vi "findNewLocation.vi"(8 "error in (no error)":errorcluster, 9 "possible \nlocations":dbl[](array[numeric]), 11 "start \nlocation":dbl[](array[numeric])) -> (0 "error out":errorcluster, 3 "new\nplatform":i32)   [LabVIEW 2017]
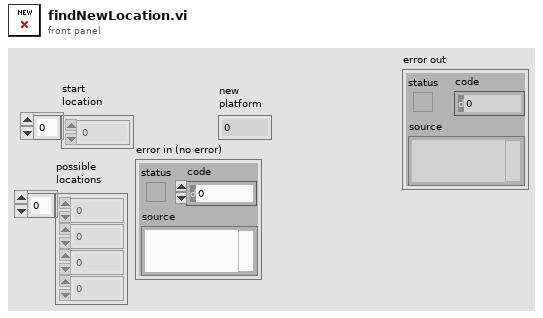
[diagram p1: front panel]
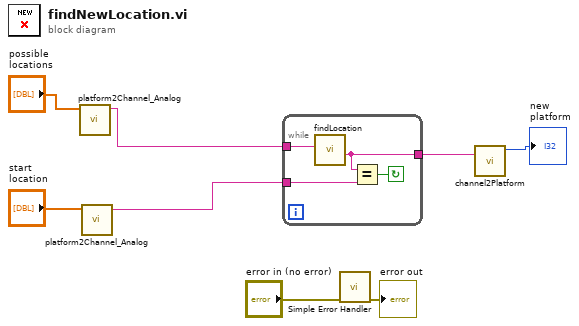
[diagram p0: block diagram]
diagram:
  n1 = call "platform2Channel_Analog.vi"("platforms"="possible \nlocations") -> ("DAQmx Channel"=w8:string)  [unwired: 10 in]
  n2 = call "platform2Channel_Analog.vi"("platforms"="start \nlocation") -> ("DAQmx Channel"=w5:string)  [unwired: 10 in]
  n3 = while {
    tunnel: w5 -> [w11]
    tunnel: [w10] -> w4
    tunnel: w8 -> [w9]
    stop <- w12 continue-if-true
    n4 = call "findLocation.vi"("DAQmx \nPhysical Channel"=w9) -> ("Animals location"=w10:string)  [unwired: 10 in]
    n5 = Equal?(x=w10, y=w11) -> (x = y?=w12:bool)
  }
  n6 = call <vilib>:"Simple Error Handler.vi"("error in (no error)"="error in (no error)") -> ("error out"=→"error out":errorcluster)  [unwired: 4 in, 4 out]
  n7 = call "channel2Platform.vi"("DAQmx \nPhysical Channel"=w4) -> ("Platform number"=→"new\nplatform":i32)  [unwired: 10 in]
